vi "IntegerMeasure.vi"(5 "EndTime":timestamp, 7 "StartTime":timestamp, 8 "error in":errorcluster, 11 "IntegerlMeasure":refnum<class "IntegerMeasure.lvclass">) -> (0 "error out":errorcluster, 3 "Passed":bool)   [LabVIEW 2020]
uses:
  ProligentResultProcessor/Measure/IntegerMeasure/IntegerMeasure.lvclass
  C:/Projects/Result Processor/src/LabVIEWResultProcessor/ProligentResultProcessor/Measure/Measure/Measure.lvclass
  ProligentResultProcessor/Measure/IntegerMeasureLimit/IntegerMeasureLimit.lvclass
  C:/Projects/Result Processor/src/LabVIEWResultProcessor/ProligentResultProcessor/Measure/RangeMeasureLimit/RangeMeasureLimit.lvclass
  C:/Projects/Result Processor/src/LabVIEWResultProcessor/ProligentResultProcessor/Measure/MeasureLimit/MeasureLimit.lvclass
  ProligentResultProcessor/Measure/RangeMeasureLimit/ComparisonType.ctl
  ProligentResultProcessor/Measure/Measure/SetStartDate.vi
  ProligentResultProcessor/Measure/Measure/SetMeasureExecutionStatus.vi
  ProligentResultProcessor/Measure/IntegerMeasure/SetValue.vi
  ProligentResultProcessor/Measure/Measure/SetComments.vi
  ProligentResultProcessor/Measure/Measure/SetMeasureId.vi
  ProligentResultProcessor/Measure/Measure/GetStartDate.vi
  ProligentResultProcessor/Measure/Measure/GetMeasureExecutionStatus.vi
  ProligentResultProcessor/Measure/IntegerMeasure/GetValue.vi
  ProligentResultProcessor/Measure/Measure/GetComments.vi
  ProligentResultProcessor/Measure/Measure/GetMeasureId.vi
  ProligentResultProcessor/Measure/Measure/GetLimit.vi
  ProligentResultProcessor/Measure/IntegerMeasureLimit/SetHigherBound.vi
  ProligentResultProcessor/Measure/IntegerMeasureLimit/SetLowerBound.vi
  ProligentResultProcessor/Measure/RangeMeasureLimit/GetComparisonType.vi
  ProligentResultProcessor/Measure/IntegerMeasureLimit/GetHigherBound.vi
  ProligentResultProcessor/Measure/IntegerMeasureLimit/GetLowerBound.vi
  ProligentResultProcessor/Measure/MeasureLimit/GetLimitExpression.vi
  ProligentResultProcessor/Measure/MeasureLimit/GetCustomData.vi
  ProligentResultProcessor/Measure/MeasureLimit/MeasureLimit.lvclass
  ProligentResultProcessor/Model/CustomData/CustomData.lvclass
  ProligentResultProcessor/Measure/RangeMeasureLimit/RangeMeasureLimit.lvclass
  ProligentResultProcessor/Measure/Measure/Measure.lvclass
  C:/Projects/Result Processor/src/LabVIEWResultProcessor/ProligentResultProcessor/Measure/IntegerMeasure/IntegerMeasure.lvclass
  C:/Projects/Result Processor/src/LabVIEWResultProcessor/ProligentResultProcessor/Measure/IntegerMeasureLimit/IntegerMeasureLimit.lvclass
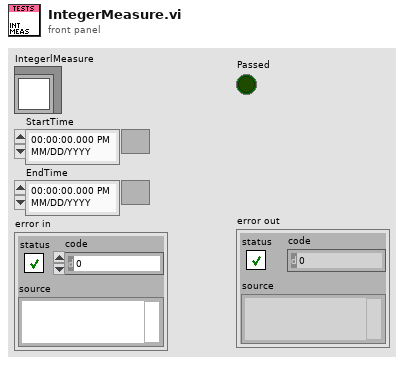
[diagram p1: front panel]
types:
  T1 = typedef "ProligentResultProcessor.lvlib/RangeMeasureLimit.lvclass/ComparisonType.ctl" = enum16{"LowerBound <= X <= HigherBound", "LowerBound < X <= HigherBound", "LowerBound <= X < HigherBound", "LowerBound < X < HigherBound", "LowerBound <= X", "LowerBound < X", "X <= HigherBound", "X < HigherBound", "X == HigherBound", "X != HigherBound", "X <= LowerBound OR HigherBound <= X", "X < LowerBound OR HigherBound <= X", "X <= LowerBound OR HigherBound < X", "X < LowerBound OR HigherBound < X"}
  T2 = enum16{"PASS", "FAIL", "NOT_COMPLETED", "ABORTED"}
  T3 = typedef "ProligentResultProcessor.lvlib/ExecutionStatus.lvclass/Value.ctl" = enum16{"PASS", "FAIL", "NOT_COMPLETED", "ABORTED"}
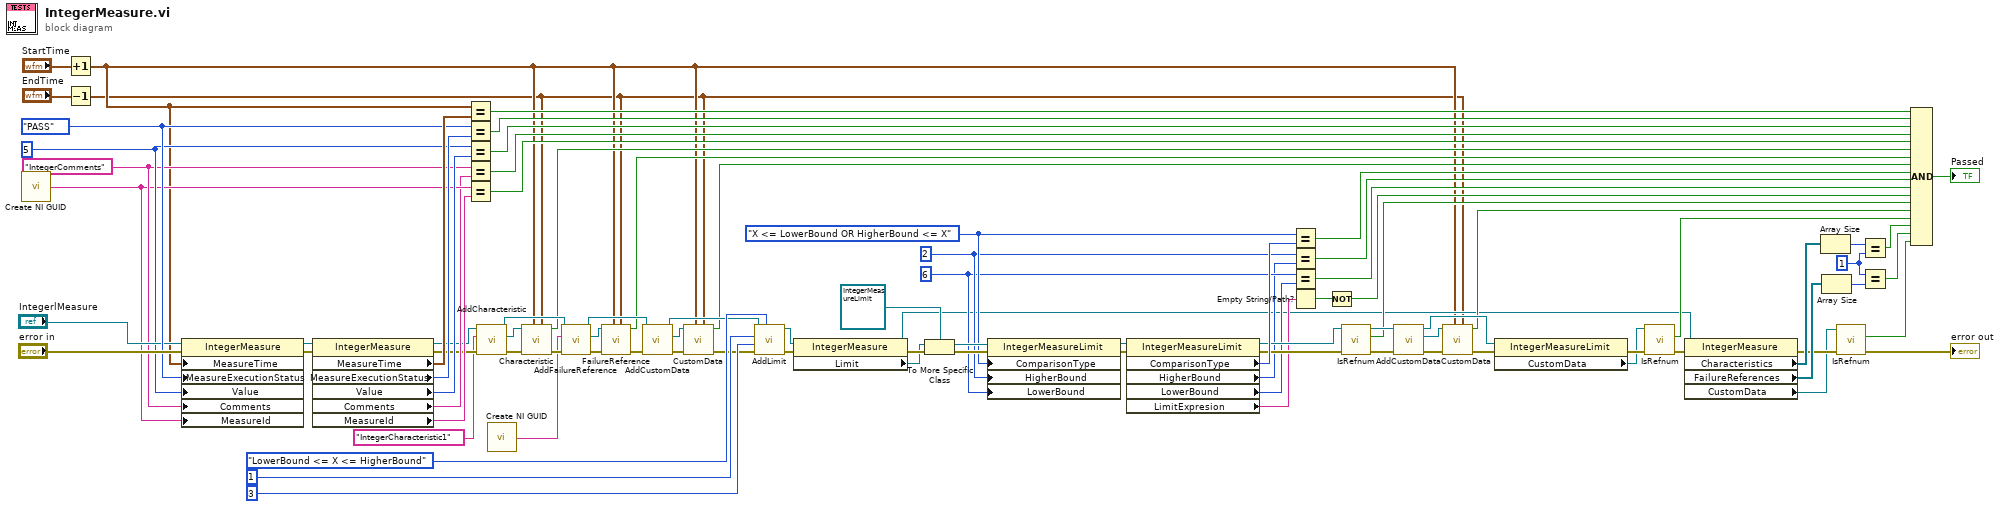
[diagram p0: block diagram]
diagram:
  w13 = 1
  w38 = "IntegerComments"
  w50 = i64 6 ("LowerBound")
  w51 = i64 2 ("LowerBound")
  w52 = ComparisonType."X <= LowerBound OR HigherBound <= X" ("ComparisonType")
  w43 = i64 5
  w80 = T2."PASS" ("ProcessRunStatus")
  n1 = call <vilib>:"Create NI GUID.vi"() -> ("NI GUID"=w37:string)
  n2 = Increment(x="StartTime") -> (x+1=w2:timestamp)
  n3 = Decrement(x="EndTime") -> (x-1=w1:timestamp)
  n4 = property class="IntegerMeasure"(reference="IntegerlMeasure", error in="error in", "MeasureTime"=w2, "MeasureExecutionStatus"=w80, "Value"=w43, "Comments"=w38, "MeasureId"=w37) -> (reference out=w91:refnum<class "IntegerMeasure.lvclass">, error out=w90:errorcluster)
  n5 = property class="IntegerMeasure"(reference=w91, error in=w90) -> (reference out=w22:refnum<class "IntegerMeasure.lvclass">, error out=w24:errorcluster, "MeasureTime"=w89:timestamp, "MeasureExecutionStatus"=w88:T3, "Value"=w87:i64, "Comments"=w36:string, "MeasureId"=w35:string)
  n6 = Equal?(x=w2, y=w89) -> (x = y?=w86:bool)
  n7 = Equal?(x=w80, y=w88) -> (x = y?=w85:bool)
  n8 = Equal?(x=w43, y=w87) -> (x = y?=w84:bool)
  n9 = Equal?(x=w38, y=w36) -> (x = y?=w40:bool)
  n10 = Equal?(x=w37, y=w35) -> (x = y?=w39:bool)
  n11 = call "AddCharacteristic.vi"("error in (no error)"=w24, "FullName"="IntegerCharacteristic1", "Measure in"=w22) -> ("error out"=w34:errorcluster, "Characteristic"=w33:refnum<class "Characteristic.lvclass">, "Measure out"=w31:refnum<class "IntegerMeasure.lvclass">)  [unwired: 6 in]
  n12 = call <vilib>:"Create NI GUID.vi"() -> ("NI GUID"=w3:string)
  n13 = call "Characteristic.vi"("EndTime"=w1, "StartTime"=w2, "error in (no error)"=w34, "Characteristic in"=w33) -> ("error out"=w32:errorcluster, "Passed"=w20:bool)  [unwired: 6 in]
  n14 = call "AddFailureReference.vi"("error in (no error)"=w32, "Id"=w3, "Measure in"=w31) -> ("error out"=w26:errorcluster, "FailureReference"=w25:refnum<class "FailureReference.lvclass">, "Measure out"=w28:refnum<class "IntegerMeasure.lvclass">)  [unwired: 6 in]
  n15 = call "FailureReference.vi"("EndTime"=w1, "StartTime"=w2, "error in"=w26, "Defect"=w25) -> ("error out"=w30:errorcluster, "Passed"=w19:bool)  [unwired: 6 in]
  n16 = call "AddCustomData.vi"("error in (no error)"=w30, "Measure in"=w28) -> ("error out"=w29:errorcluster, "CustomData"=w27:refnum<class "CustomData.lvclass">, "Measure out"=w21:refnum<class "IntegerMeasure.lvclass">)  [unwired: 7 in]
  n17 = call "CustomData.vi"("EndTime"=w1, "StartTime"=w2, "error in"=w29, "CustomData"=w27) -> ("error out"=w23:errorcluster, "Passed"=w18:bool)  [unwired: 6 in]
  n18 = call "AddLimit.vi"("ComparisonType"=ComparisonType."LowerBound <= X <= HigherBound", "error in"=w23, "HigherBond"=i64 3 ("LowerBound"), "LowerBound"=i64 1, "IntergerMeasure in"=w21) -> ("error out"=w74:errorcluster, "IntergerMeasure out"=w79:refnum<class "IntegerMeasure.lvclass">)  [unwired: 4 in, 1 out]
  n19 = property class="IntegerMeasure"(reference=w79, error in=w74) -> (reference out=w16:refnum<class "IntegerMeasure.lvclass">, error out=w78:errorcluster, "Limit"=w75:refnum<class "MeasureLimit.lvclass">)
  n20 = To More Specific Class(target class=refnum<class "IntegerMeasureLimit.lvclass"> refnum ("ProligentResultProcessor:IntegerMeasureLimit"), reference=w75, error in=w78) -> (specific class reference=w76:refnum<class "IntegerMeasureLimit.lvclass">, error out=w77:errorcluster)
  n21 = property class="IntegerMeasureLimit"(reference=w76, error in=w77, "ComparisonType"=w52, "HigherBound"=w51, "LowerBound"=w50) -> (reference out=w73:refnum<class "IntegerMeasureLimit.lvclass">, error out=w72:errorcluster)
  n22 = property class="IntegerMeasureLimit"(reference=w73, error in=w72) -> (reference out=w64:refnum<class "IntegerMeasureLimit.lvclass">, error out=w69:errorcluster, "ComparisonType"=w71:T1, "HigherBound"=w49:i64, "LowerBound"=w48:i64, "LimitExpresion"=w53:string)
  n23 = Equal?(x=w52, y=w71) -> (x = y?=w47:bool)
  n24 = Equal?(x=w51, y=w49) -> (x = y?=w46:bool)
  n25 = Equal?(x=w50, y=w48) -> (x = y?=w45:bool)
  n26 = Empty String/Path?(string/path=w53) -> (empty?=w70:bool)
  n27 = Not(x=w70) -> (.not. x?=w41:bool)
  n28 = call "IsRefnum.vi"("error in"=w69, "MeasureLimit in"=w64) -> ("error out"=w65:errorcluster, "IsRefnum"=w62:bool, "MeasureLimit out"=w63:refnum<class "IntegerMeasureLimit.lvclass">)  [unwired: 7 in]
  n29 = call "AddCustomData.vi"("error in"=w65, "MeasureLimit in"=w63) -> ("error out"=w60:errorcluster, "CustomData"=w58:refnum<class "CustomData.lvclass">, "MeasureLimit out"=w61:refnum<class "IntegerMeasureLimit.lvclass">)  [unwired: 7 in]
  n30 = call "CustomData.vi"("EndTime"=w1, "StartTime"=w2, "error in"=w60, "CustomData"=w58) -> ("error out"=w59:errorcluster, "Passed"=w57:bool)  [unwired: 6 in]
  n31 = property class="IntegerMeasureLimit"(reference=w61, error in=w59) -> (error out=w68:errorcluster, "CustomData"=w67:refnum<class "CustomData.lvclass">)  [unwired: 1 out]
  n32 = call "IsRefnum.vi"("error in"=w68, "CustomDataType in"=w67) -> ("error out"=w17:errorcluster, "IsRefnum"=w66:bool)  [unwired: 7 in, 1 out]
  n33 = property class="IntegerMeasure"(reference=w16, error in=w17) -> (error out=w8:errorcluster, "Characteristics"=w10:refnum<class "Characteristic.lvclass">[], "FailureReferences"=w9:refnum<class "FailureReference.lvclass">[], "CustomData"=w6:refnum<class "CustomData.lvclass">)  [unwired: 1 out]
  n34 = Array Size(array=w10) -> (size(s)=w15:i32)
  n35 = Array Size(array=w9) -> (size(s)=w14:i32)
  n36 = call "IsRefnum.vi"("error in"=w8, "CustomDataType in"=w6) -> ("error out"=→"error out":errorcluster, "IsRefnum"=w5:bool)  [unwired: 7 in, 1 out]
  n37 = Equal?(x=w15, y=w13) -> (x = y?=w12:bool)
  n38 = Equal?(x=w13, y=w14) -> (x = y?=w11:bool)
  n39 = Compound Arithmetic op=AND(w86, w85, w84, w40, w39, w20, w19, w18, w47, w46, w45, w41, w62, w57, w66, w12, w11, w5) -> (→"Passed":bool)
